vi "Init.vi"(8 "error in (no error)":errorcluster) -> (0 "error out":errorcluster, 3 "Module IDs":i32[](array[numeric]), 4 "First? (all)":bool[](array[boolean]), 5 "Instances Names":string[](array[string]))   [LabVIEW 2020, in "ExampleClone.lvlib" / "Clone Registration.lvlib"]
doc: "Initialize the cloneable module registry.\n____\nHAMPEL SOFTWARE ENGINEERING v2.6.0 (2023-12-19 10:54)"
uses:
  Clone Registration.lvlib
  Action--enum.ctl
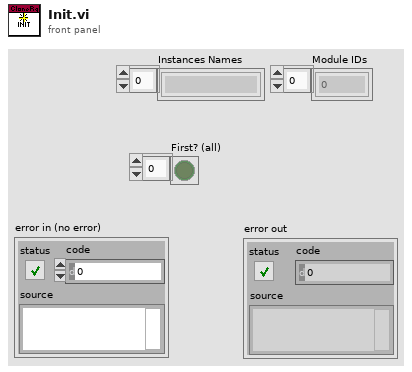
[diagram p1: front panel]
types:
  T1 = typedef "ExampleClone.lvlib/Clone Registration.lvlib/Action--enum.ctl" = enum16{"Init", "Add Instance", "Remove Instance", "List Instances", "Is First?"}
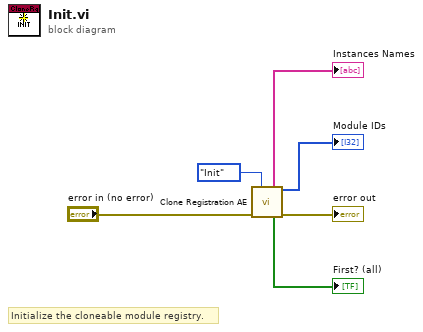
[diagram p0: block diagram]
diagram:
  # "Initialize the cloneable module registry."
  n1 = call "Clone Registration AE.vi"("Action"=Action--enum."Init", "error in (no error)"="error in (no error)") -> ("Instances Names"=→"Instances Names":string[], "Module IDs"=→"Module IDs":i32[], "First? (all)"=→"First? (all)":bool[], "error out"=→"error out":errorcluster)  [unwired: 5 in, 5 out]
